vi "ERRMSGdll_Test.vi"(8 "error in (no error)":errorcluster) -> (0 "error out":errorcluster caption="Returned error out", 3 "Passed?":bool)   [LabVIEW 2016]
panel:
  out "Actual Error Code":i32
  out "Actual Error Text":string
  out "Actual Error out":errorcluster caption="Generated error out"
  out "ierr":i32
  out "herr":string
  out "herr_length":i32
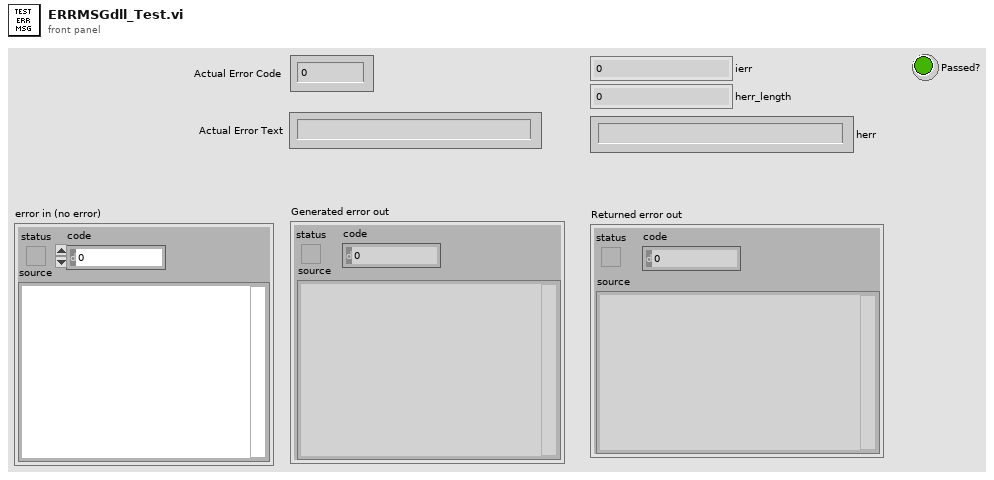
[diagram p1: front panel]
types:
  T1 = cluster{"kFlag":i32, "ierr":i32, "herr":string, "herr length":i32, "hFlag length":i32}
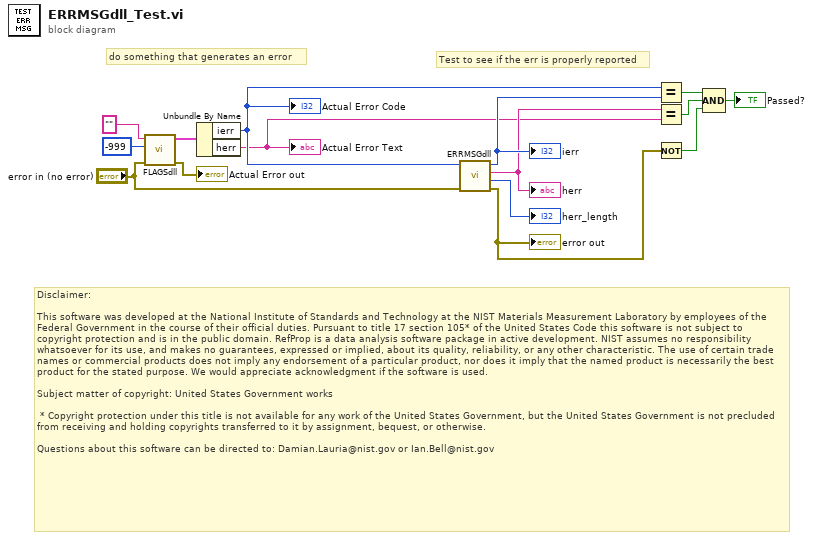
[diagram p0: block diagram]
diagram:
  # "Disclaimer:\n\nThis software was developed at the National Institute of Standards and Technology at the NIST Materials Measurement Laboratory by employees of the Federal Government in the course of their official duties. Pursuant to title 17 section 105* of the United States Code this software is not subject to copyright protection and is in the public domain. RefProp is a data analysis software package in active development. NIST assumes no responsibility whatsoever for its use, and makes no guarantees, expressed or implied, about its quality, reliability, or any other characteristic. The use of certain trade names or commercial products does not imply any endorsement of a particular product, nor does it imply that the named product is necessarily the best product for the stated purpose. We would appreciate acknowledgment if the software is used.\n \nSubject matter of copyright: United States Government works\n  \n * Copyright protection under this title is not available for any work of the United States Government, but the United States Government is not precluded from receiving and holding copyrights transferred to it by assignment, bequest, or otherwise.\n\nQuestions about this software can be directed to: Damian.Lauria@nist.gov or Ian.Bell@nist.gov"
  # "Test to see if the err is properly reported"
  # "do something that generates an error"
  n1 = call "FLAGSdll.vi"("error in (no error)"="error in (no error)", "jFlag"=-999, "hFlag"="") -> ("error out"=→"Actual Error out":errorcluster, "Outputs"=w3:T1)  [unwired: 7 in]
  n2 = Unbundle By Name(w3) -> ("ierr"=w2:i32, "herr"=w1:string)
  "Actual Error Text" <- w1
  "Actual Error Code" <- w2
  n3 = call "ERRMSGdll.vi"("error in (no error)"="error in (no error)", "ierr in"=w2) -> ("error out"=w6:errorcluster, "herr_length"=→"herr_length":i32, "herr"=w11:string, "ierr"=w12:i32)  [unwired: 6 in]
  "error out" <- w6
  "herr" <- w11
  "ierr" <- w12
  n4 = Equal?(x=w2, y=w12) -> (x = y?=w9:bool)
  n5 = Equal?(x=w11, y=w1) -> (x = y?=w8:bool)
  n6 = Not(x=w6) -> (.not. x?=w5:bool)
  n7 = Compound Arithmetic op=AND(w9, w8, w5) -> (→"Passed?":bool)
